vi "test Is Anchor ID Unique True.vi"(8 "error in (no error)":errorcluster, 11 "TestCase in":refnum<class "Utility VIs tests.lvclass">) -> (0 "error out":errorcluster, 3 "TestCase out":refnum<class "Utility VIs tests.lvclass">)   [LabVIEW 2014, in "Utility VIs tests.lvclass"]
uses:
  Utility VIs tests.lvclass
  SPLAT/Anchor/Anchor.lvclass
  <vilib>/addons/_JKI Toolkits/VI Tester/TestCase.llb/TestCase.lvclass
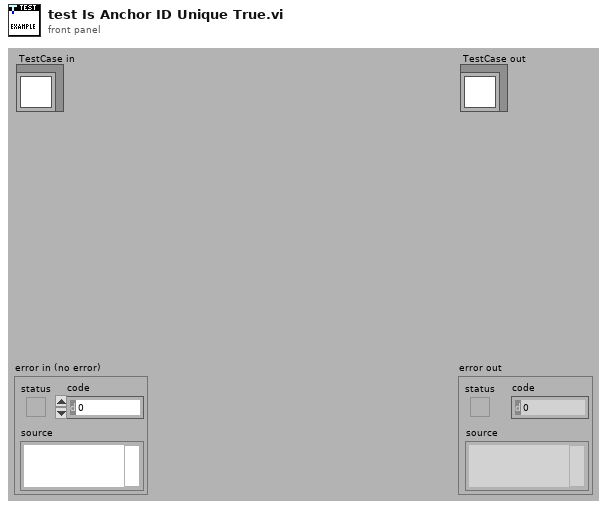
[diagram p1: front panel]
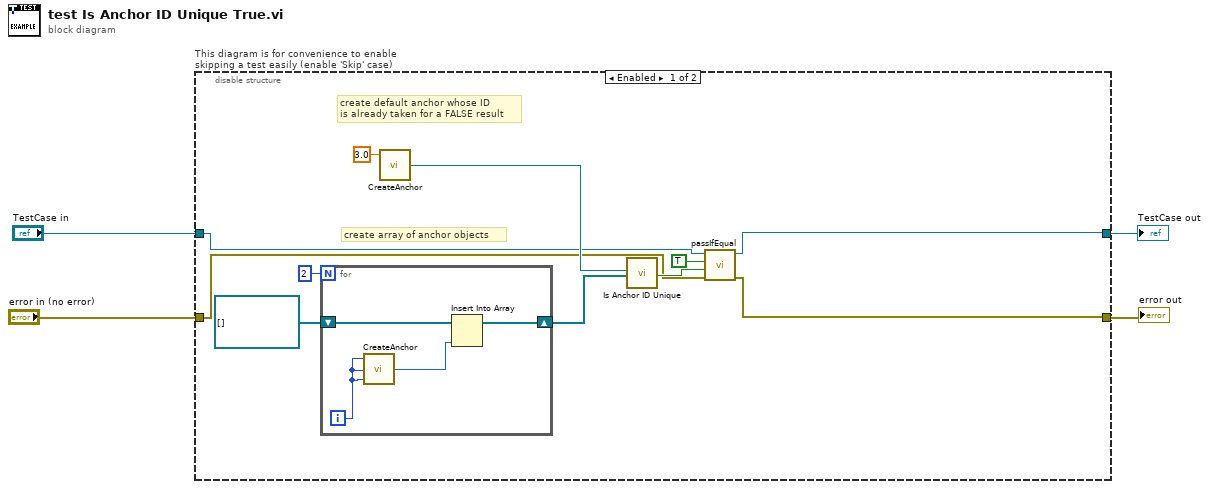
[diagram p0: block diagram]
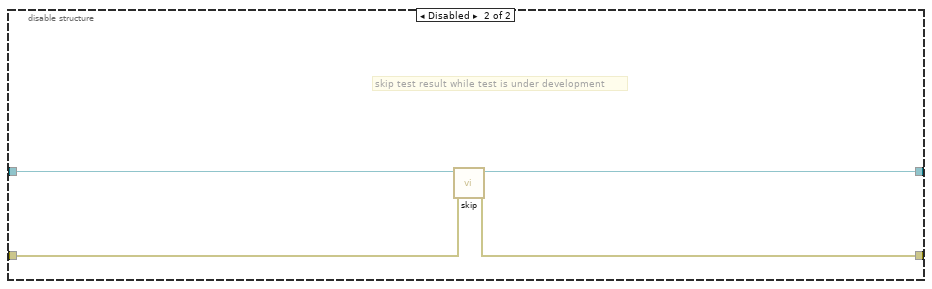
[diagram p2: hidden frame]
diagram:
  n1 = disable-structure "This diagram is for convenience to enable skipping a test easily (enable 'Skip' case)" shown="Enabled" {
    disable-tunnel: "TestCase in" -> [w8 w23]
    disable-tunnel: [w10 w21] -> w1
    disable-tunnel: [w9 w22] -> w3
    disable-tunnel: "error in (no error)" -> [w7 w20]
    frame Enabled {
      # "create default anchor whose ID \nis already taken for a FALSE result"
      # "create array of anchor objects"
      n2 = for {
        N: 2 -> [_]
        shift-right: [w18] -> w14
        shift-left: refnum<class "Anchor.lvclass">[] [] -> [w19]
        i -> [w17]
        n3 = call "CreateAnchor.vi"("Anchor Y"=w17, "Anchor X"=w17, "Anchor ID"=w17) -> ("Anchor Out"=w16:refnum<class "Anchor.lvclass">)
        n4 = Insert Into Array(array=w19, new element=w16) -> (w18:refnum<class "Anchor.lvclass">[])  [unwired: 1 in]
      }
      n5 = call "CreateAnchor.vi"("Anchor ID"=3.0) -> ("Anchor Out"=w13:refnum<class "Anchor.lvclass">)  [unwired: 2 in]
      n6 = call "Is Anchor ID Unique.vi"("Anchor.lvclass"=w13, "Input AnchorArray"=w14) -> ("Is unique?"=w12:bool)  [unwired: 17 in]
      n7 = call-dynamic "passIfEqual.vi"("error in (no error)"=w7, "y"=w12, "x"=TRUE, "TestCase in"=w8) -> ("error out"=w9:errorcluster, "TestCase out"=w10:refnum<class "Utility VIs tests.lvclass">)  [unwired: 6 in]
    }
    frame Disabled {
      # "skip test result while test is under development"
      n8 = call <vilib>:"skip.vi"("error in (no error)"=w20, "TestCase in"=w23) -> ("error out"=w22:errorcluster, "TestCase out"=w21:refnum<class "Utility VIs tests.lvclass">)  [unwired: 8 in]
    }
  }
  "error out" <- w3
  "TestCase out" <- w1
